vi "Read Error.vi"(8 "error in (no error)":errorcluster, 11 "ErrorMessage.lvclass in":refnum<class "ErrorMessage.lvclass">) -> (0 "error out":errorcluster, 2 "Error":errorcluster, 3 "ErrorMessage.lvclass out":refnum<class "ErrorMessage.lvclass">)   [LabVIEW 2011, in "Messenging.lvlib" / "ErrorMessage.lvclass"]
uses:
  ErrorMessage.lvclass
  ErrorMessage.lvclass/ErrorMessage.ctl
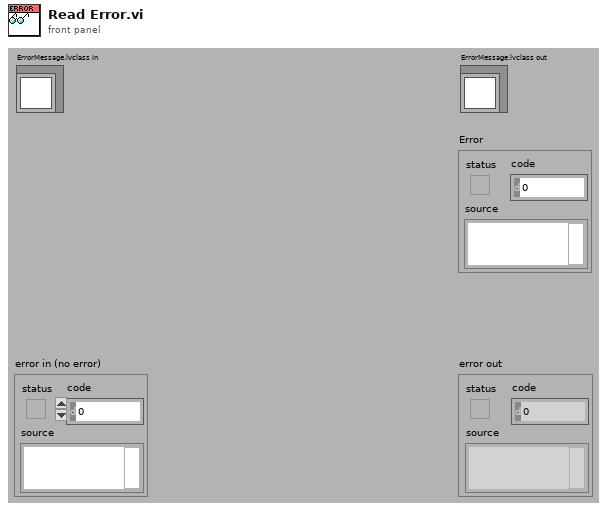
[diagram p1: front panel]
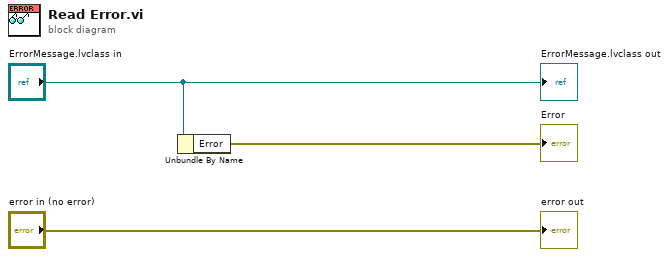
[diagram p0: block diagram]
diagram:
  n1 = Unbundle By Name("ErrorMessage.lvclass in") -> ("Error"=→"Error":errorcluster)
  "error out" <- "error in (no error)"
  "ErrorMessage.lvclass out" <- "ErrorMessage.lvclass in"
